vi "Encoder for velocity - Copy.vi"() -> ()   [LabVIEW 2020]
uses:
  <vilib>/DAQmx/read.llb/DAQmx Read (Counter DBL 1Chan 1Samp).vi
  <vilib>/DAQmx/read.llb/DAQmx Read (Counter U32 1Chan 1Samp).vi
  <vilib>/DAQmx/miscellaneous.llb/DAQmx Fill In Error Info.vi
  <vilib>/DAQmx/create/channels.llb/DAQmx Create Channel (CI-Count Edges).vi
  <vilib>/ptbypt/NI_PtbyPt.lvlib
  <resource>/objmgr/daqmx.rc
panel:
  out "Waveform Chart for velocity":dbl(graph)
  in  "Edge?":bool
  in  "stop":bool
  out "edge":u32
  in  "error in":errorcluster
  out "frequence":dbl format="%0.2f"
  in  "radius":dbl
  in  "counts per Revolution":dbl=2048.0
  out "velocity":dbl
  out "Waveform Chart 2":dbl[](graph)
  out "largest Velocity":dbl
  in  "sampling point":i32=500
  out "trigger":bool
  in  "Record start value":dbl=100.0
  out "Waveform Chart for frequency":dbl(graph)
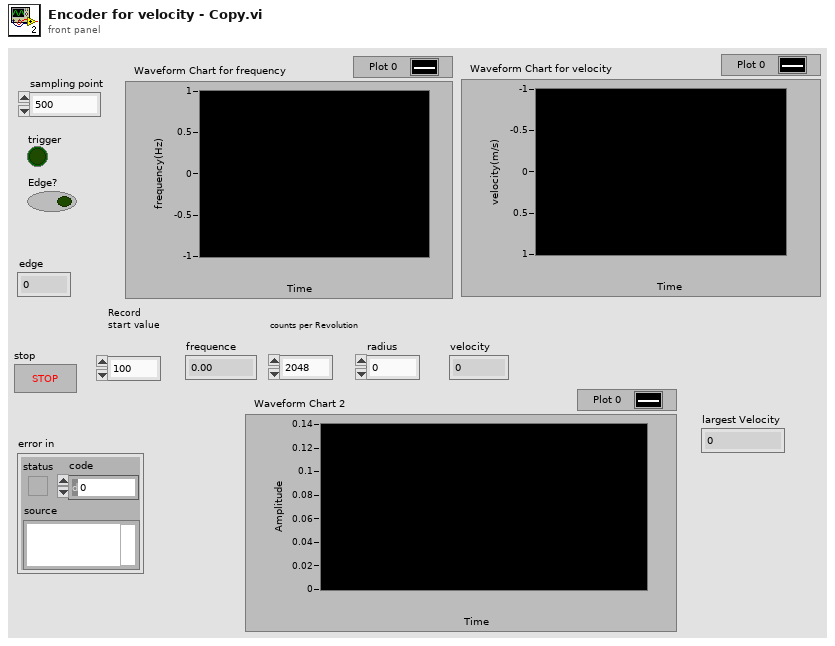
[diagram p1: front panel]
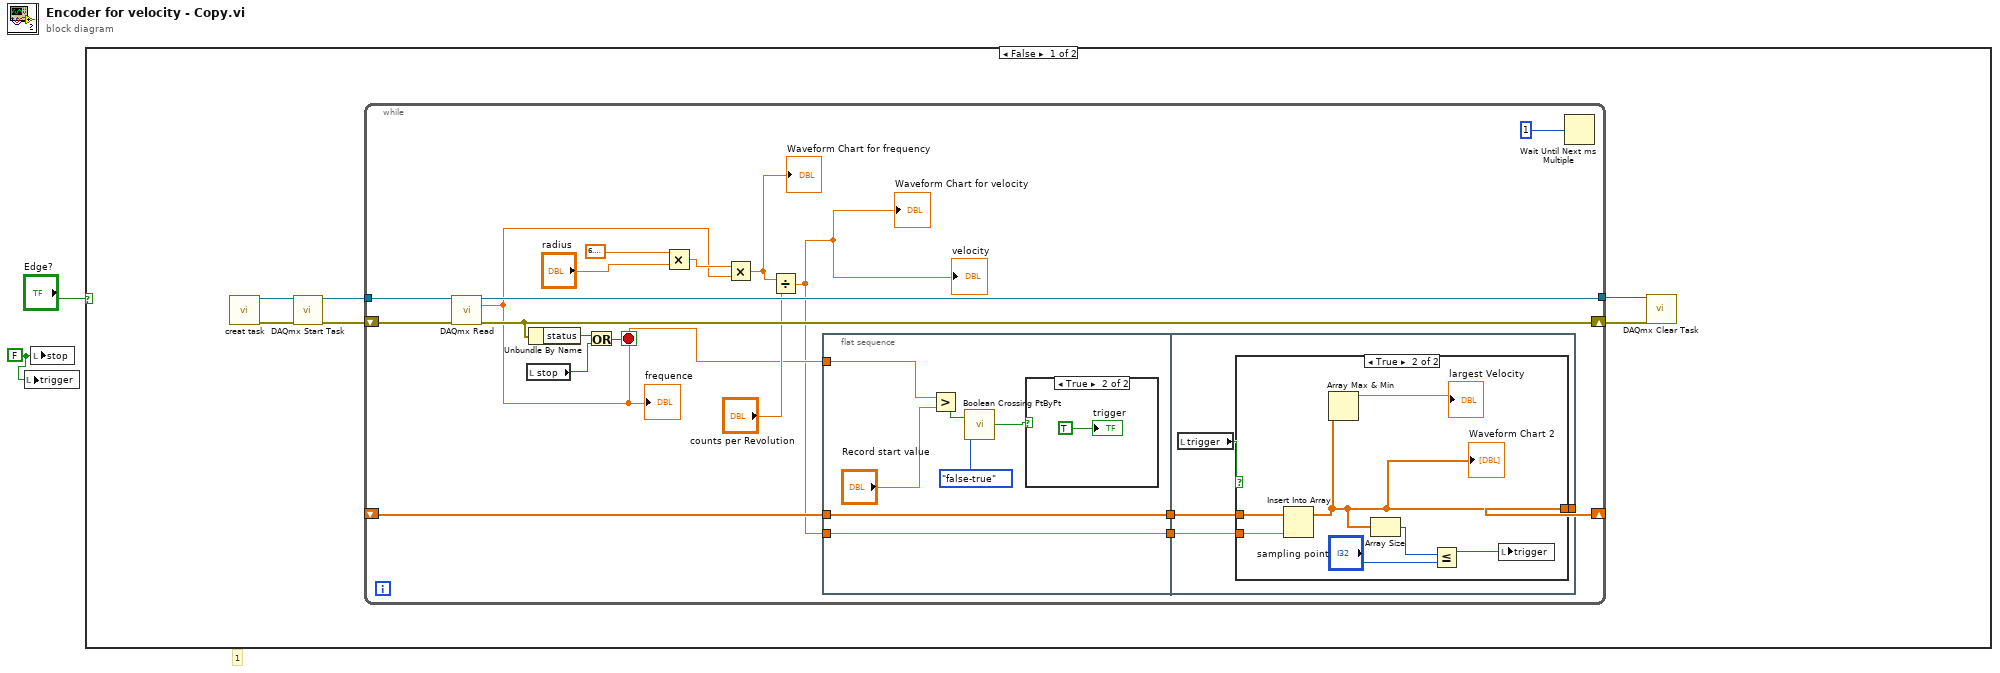
[diagram p0: block diagram]
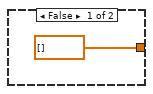
[diagram p3: hidden frame]
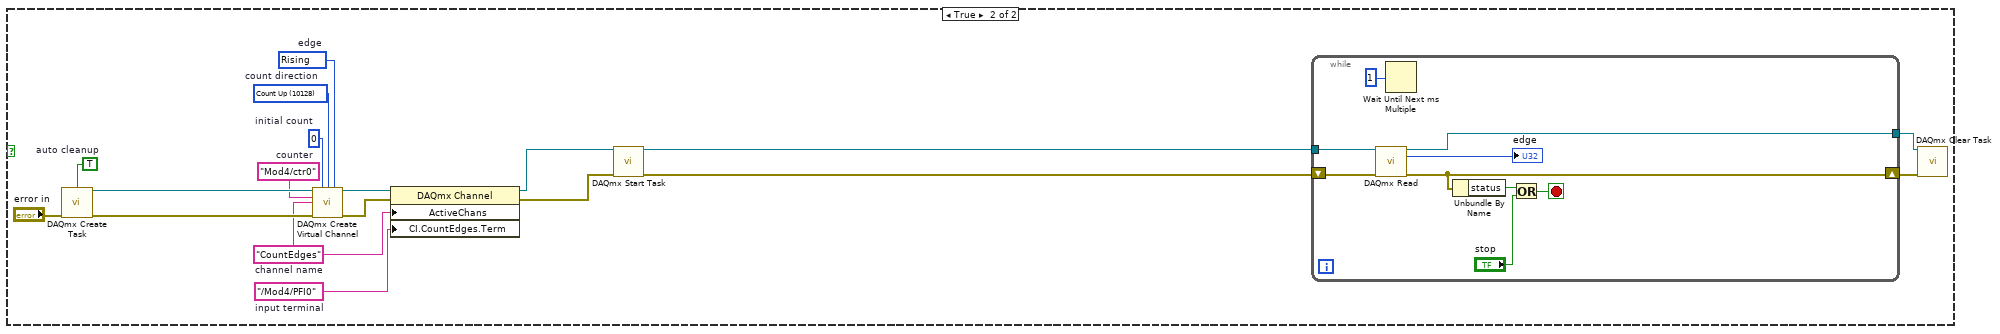
[diagram p4: hidden frame]
diagram:
  w1 = FALSE ("stop")
  # "1"
  n1 = local write "trigger"(w1) -> ()
  n2 = local write "stop"(w1) -> ()
  n3 = case shown="False" "Edge?" {
    frame False {
      n4 = call "creat task.vi"() -> ("error out"=w8:errorcluster, "task out"=w7:refnum<k21>)  [unwired: 10 in]
      n5 = call <vilib>:"DAQmx Start Task.vi"("task/channels in"=w7, "error in"=w8) -> ("task out"=w3:refnum<k21>, "error out"=w4:errorcluster)  [unwired: 12 in]
      n6 = while {
        tunnel: w3 -> [w27]
        tunnel: [w25] -> w6
        shift-right: [w24] -> w5
        shift-left: w4 -> [w26]
        shift-right: [w16] -> _
        shift-left: _ -> [w15]
        stop <- w22 stop-if-true
        n7 = call-poly <vilib>:"DAQmx Read.vi"("task/channels in"=w27, "error in"=w26) -> ("task out"=w25:refnum<k21>, "data"=w12:dbl, "error out"=w24:errorcluster)  [unwired: 11 in]
        "frequence" <- w12
        n8 = local read "stop"() -> (w17:bool)
        n9 = Unbundle By Name(w24) -> ("status"=w23:bool)
        n10 = Or(x=w23, y=w17) -> (x .or. y?=w22:bool)
        n11 = Multiply(x=6.283185307179586, y="radius") -> (x*y=w19:dbl)
        n12 = Multiply(x=w19, y=w12) -> (x*y=w10:dbl)
        "Waveform Chart for frequency" <- w10
        n13 = Divide(x=w10, y="counts per Revolution") -> (x/y=w9:dbl)
        "velocity" <- w9
        "Waveform Chart for velocity" <- w9
        n14 = flat-sequence {
          tunnel: w15 -> [w33]
          tunnel: w9 -> [w34]
          tunnel: [w34] -> w14
          tunnel: [w33] -> w13
          tunnel: w12 -> [w30]
          tunnel: [w38] -> w16
          tunnel: w14 -> [w39]
          tunnel: w13 -> [w37]
          frame #0 {
            n15 = Greater?(x=w30, y="Record start value") -> (0:w31:bool)
            n16 = call <vilib>:"Boolean Crossing PtByPt.vi"("direction"=enum16{"either", "false-true", "true-false"}."false-true", "input"=w31) -> ("crossing"=w29:bool)  [unwired: 1 in]
            n17 = case shown="True" w29 {
              frame False {
              }
              frame True {
                "trigger" <- TRUE ("x >= y?")
              }
            }
          }
          frame #1 {
            n18 = local read "trigger"() -> (w36:bool)
            n19 = case shown="True" w36 {
              tunnel: w39 -> [_ w47]
              tunnel: [dbl[] [] w43] -> w38
              tunnel: w37 -> [_ w46]
              frame False {
              }
              frame True {
                n20 = Insert Into Array(array=w46, new element=w47) -> (w43:dbl[])  [unwired: 1 in]
                "Waveform Chart 2" <- w43
                n21 = Array Max & Min(array=w43) -> (max value=→"largest Velocity":dbl)  [unwired: 3 out]
                n22 = Array Size(array=w43) -> (size(s)=w45:i32)
                n23 = Less Or Equal?(x=w45, y="sampling point") -> (x <= y?=w41:bool)
                n24 = local write "trigger"(w41) -> ()
              }
            }
          }
        }
        n25 = Wait Until Next ms Multiple(millisecond multiple=u32 1) -> ()  [unwired: 1 out]
      }
      n26 = call <vilib>:"DAQmx Clear Task.vi"("task in"=w6, "error in"=w5) -> ()  [unwired: 13 in, 1 out]
    }
    frame True {
      w50 = "/Mod4/PFI0"  # input terminal
      w53 = 10280 items=["Rising"=10280, "Falling"=10171]  # edge
      w54 = 10128 items=["Count Up"=10128, "Count Down"=10124, "Externally Controlled"=10326]  # count direction
      w55 = u32 0  # initial count
      w51 = "CountEdges"  # channel name
      w57 = "Mod4/ctr0"  # counter
      w59 = TRUE  # auto cleanup
      n27 = call <vilib>:"DAQmx Create Task.vi"("auto cleanup"=w59, "error in"="error in") -> ("task out"=w58:refnum<k21>, "error out"=w60:errorcluster)  [unwired: 12 in]
      n28 = call-poly <vilib>:"DAQmx Create Virtual Channel.vi"("task in"=w58, "initial count"=w55, "count direction"=w54, "edge"=w53, "counter"=w57, "name to assign"=w51, "error in"=w60) -> ("task out"=w52:refnum<k21>, "error out"=w56:errorcluster)  [unwired: 7 in]
      n29 = property class="DAQmx Channel"(reference=w52, error in=w56, "ActiveChans"=w51, "CI.CountEdges.Term"=w50) -> (reference out=w49:refnum<k21>, error out=w48:errorcluster)
      n30 = call <vilib>:"DAQmx Start Task.vi"("task/channels in"=w49, "error in"=w48) -> ("task out"=w65:refnum<k21>, "error out"=w64:errorcluster)  [unwired: 12 in]
      n31 = while {
        tunnel: w65 -> [w74]
        tunnel: [w72] -> w62
        shift-right: [w70] -> w63
        shift-left: w64 -> [w73]
        stop <- w68 stop-if-true
        n32 = call-poly <vilib>:"DAQmx Read.vi"("task/channels in"=w74, "error in"=w73) -> ("task out"=w72:refnum<k21>, "data"=→"edge":u32, "error out"=w70:errorcluster)  [unwired: 11 in]
        n33 = Wait Until Next ms Multiple(millisecond multiple=u32 1) -> ()  [unwired: 1 out]
        n34 = Unbundle By Name(w70) -> ("status"=w71:bool)
        n35 = Or(x=w71, y="stop") -> (x .or. y?=w68:bool)
      }
      n36 = call <vilib>:"DAQmx Clear Task.vi"("task in"=w62, "error in"=w63) -> ()  [unwired: 13 in, 1 out]
    }
  }
